vi "tra25cc_config.vi"(4 "speed_xyz":cluster{"speed_z":dbl, "speed_xy":dbl}={"speed_z"=0.4, "speed_xy"=0.4}, 6 "tracking mode":i32=1, 8 "error in (no error)":errorcluster, 11 "conn_xyz_in":T2) -> (0 "error out":errorcluster, 3 "conn_xyz_out":T1)   [LabVIEW 2014]
uses:
  \\CL3-USR4\usr4/F103625/Scanner_v3_current/src/Stage_xyz/Dll/Newport.CONEXCC.CommandInterface.dll
  Dll/Newport.CONEXCC.CommandInterface.dll
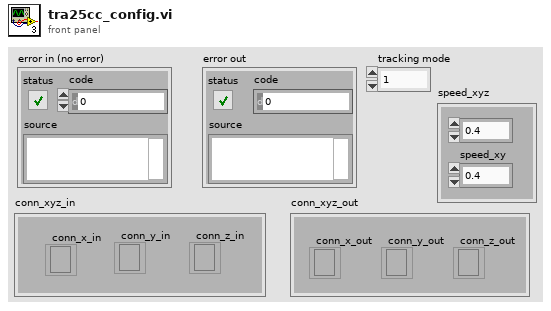
[diagram p1: front panel]
types:
  T1 = cluster{"conn_x_out":refnum<k24>, "conn_y_out":refnum<k24>, "conn_z_out":refnum<k24>}
  T2 = cluster{"conn_x_in":refnum<k24>, "conn_y_in":refnum<k24>, "conn_z_in":refnum<k24>}
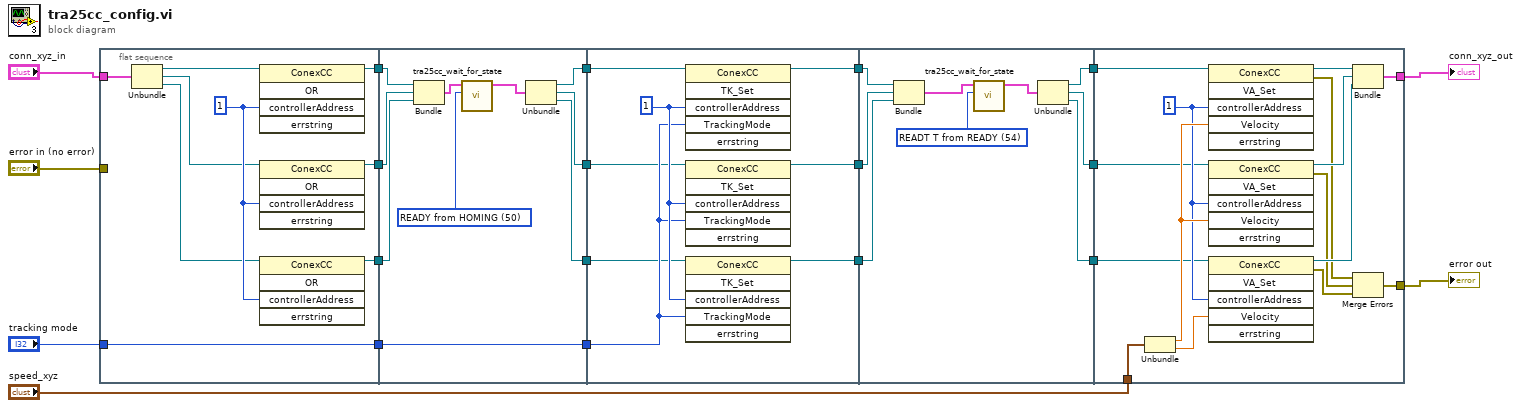
[diagram p0: block diagram]
diagram:
  n1 = flat-sequence {
    tunnel: "tracking mode" -> [w29]
    tunnel: "conn_xyz_in" -> [w24]
    tunnel: "error in (no error)" -> [_]
    tunnel: [w29] -> w14
    tunnel: [w23] -> w13
    tunnel: [w22] -> w12
    tunnel: [w21] -> w11
    tunnel: w14 -> [w39]
    tunnel: [w39] -> w10
    tunnel: w13 -> [w34]
    tunnel: [w33] -> w9
    tunnel: w12 -> [w35]
    tunnel: [w32] -> w8
    tunnel: w11 -> [w36]
    tunnel: [w31] -> w7
    tunnel: w10 -> [w46]
    tunnel: w9 -> [w45]
    tunnel: [w40] -> w15
    tunnel: w8 -> [w44]
    tunnel: [w41] -> w16
    tunnel: w7 -> [w43]
    tunnel: [w42] -> w17
    tunnel: w15 -> [w53]
    tunnel: [w50] -> w6
    tunnel: w16 -> [w52]
    tunnel: [w49] -> w5
    tunnel: w17 -> [w51]
    tunnel: [w48] -> w4
    tunnel: w6 -> [w59]
    tunnel: w5 -> [w58]
    tunnel: w4 -> [w57]
    tunnel: "speed_xyz" -> [w60]
    tunnel: [w71] -> w3
    tunnel: [w70] -> w2
    frame #0 {
      w28 = 1 ("controllerAddress")
      n2 = Unbundle(w24) -> ("conn_x_in"=w25:refnum<k24>, "conn_y_in"=w26:refnum<k24>, "conn_z_in"=w27:refnum<k24>)
      n3 = invoke class="ConexCC" method="OR"(reference=w25, "controllerAddress"=w28) -> (reference out=w23:refnum<k24>)  [unwired: 3 in, 4 out]
      n4 = invoke class="ConexCC" method="OR"(reference=w26, "controllerAddress"=w28) -> (reference out=w22:refnum<k24>)  [unwired: 3 in, 4 out]
      n5 = invoke class="ConexCC" method="OR"(reference=w27, "controllerAddress"=w28) -> (reference out=w21:refnum<k24>)  [unwired: 3 in, 4 out]
    }
    frame #1 {
      w30 = u32 50 items=["READY from HOMING"=50] ("state_to_wait")
      n6 = Bundle("conn_x_in"=w34, "conn_y_in"=w35, "conn_z_in"=w36) -> (w37:T2)  [unwired: 1 in]
      n7 = call "tra25cc_wait_for_state.vi"("state_to_wait"=w30, "conn_xyz_in"=w37) -> ("conn_xyz_out"=w38:T1)  [unwired: 7 in, 2 out]
      n8 = Unbundle(w38) -> ("conn_x_out"=w33:refnum<k24>, "conn_y_out"=w32:refnum<k24>, "conn_z_out"=w31:refnum<k24>)
    }
    frame #2 {
      w47 = 1 ("controllerAddress")
      n9 = invoke class="ConexCC" method="TK_Set"(reference=w45, "controllerAddress"=w47, "TrackingMode"=w46) -> (reference out=w40:refnum<k24>)  [unwired: 3 in, 5 out]
      n10 = invoke class="ConexCC" method="TK_Set"(reference=w44, "controllerAddress"=w47, "TrackingMode"=w46) -> (reference out=w41:refnum<k24>)  [unwired: 3 in, 5 out]
      n11 = invoke class="ConexCC" method="TK_Set"(reference=w43, "controllerAddress"=w47, "TrackingMode"=w46) -> (reference out=w42:refnum<k24>)  [unwired: 3 in, 5 out]
    }
    frame #3 {
      w54 = u32 54 items=["READY from HOMING"=50, "READT T from READY"=54] ("state_to_wait")
      n12 = Bundle("conn_x_out"=w53, "conn_y_out"=w52, "conn_z_out"=w51) -> (w55:T1)  [unwired: 1 in]
      n13 = call "tra25cc_wait_for_state.vi"("state_to_wait"=w54, "conn_xyz_in"=w55) -> ("conn_xyz_out"=w56:T1)  [unwired: 7 in, 2 out]
      n14 = Unbundle(w56) -> ("conn_x_out"=w50:refnum<k24>, "conn_y_out"=w49:refnum<k24>, "conn_z_out"=w48:refnum<k24>)
    }
    frame #4 {
      w67 = 1 ("controllerAddress")
      n15 = Unbundle(w60) -> ("speed_z"=w68:dbl, "speed_xy"=w69:dbl)
      n16 = invoke class="ConexCC" method="VA_Set"(reference=w59, "controllerAddress"=w67, "Velocity"=w68) -> (reference out=w66:refnum<k24>, error out=w63:errorcluster)  [unwired: 3 in, 4 out]
      n17 = invoke class="ConexCC" method="VA_Set"(reference=w58, "controllerAddress"=w67, "Velocity"=w68) -> (reference out=w65:refnum<k24>, error out=w62:errorcluster)  [unwired: 3 in, 4 out]
      n18 = invoke class="ConexCC" method="VA_Set"(reference=w57, "controllerAddress"=w67, "Velocity"=w69) -> (reference out=w64:refnum<k24>, error out=w61:errorcluster)  [unwired: 3 in, 4 out]
      n19 = Bundle("conn_x_out"=w66, "conn_y_out"=w65, "conn_z_out"=w64) -> (w71:T1)  [unwired: 1 in]
      n20 = Merge Errors(w63, w62, w61) -> (w70:errorcluster)
    }
  }
  "error out" <- w2
  "conn_xyz_out" <- w3
